vi "GetALL_TAGs.vi"(8 "error in (no error)":errorcluster, 11 "FAMM in":refnum<class "FAMM.lvclass">) -> (0 "error out":errorcluster, 2 "TAGs":string[](array[string]), 3 "FAMM out":refnum<class "FAMM.lvclass">)   [LabVIEW 2014, in "FAMM.lvclass"]
doc: "Read all TAGs"
uses:
  FAMM.lvclass
  FAMM.lvclass/FAMM.ctl
  Common/controls/GlobalClassRefs.vi
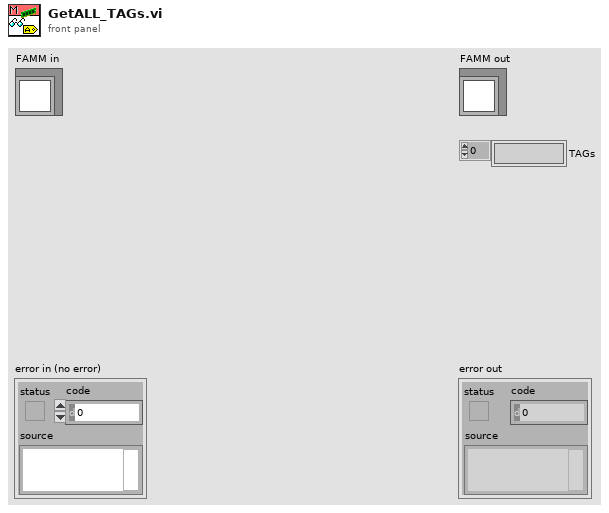
[diagram p1: front panel]
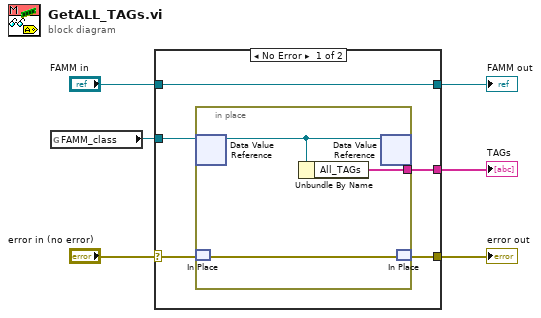
[diagram p0: block diagram]
diagram:
  n1 = global read "GlobalClassRefs.vi" "FAMM_class"() -> (w1:refnum<data-value>)
  n2 = case shown="No Error" "error in (no error)" {
    selector: "error in (no error)" -> [w9 w15]
    tunnel: [w8 w15] -> w5
    tunnel: [w11 w16] -> w3
    tunnel: "FAMM in" -> [w11 w16]
    tunnel: [w10 _] -> w2
    tunnel: w1 -> [w7 _]
    frame No Error {
      n3 = in-place {
        in-place-border: [w14] -> w10
        n4 = in-place-dvr #1(w7) -> (w12:refnum<class "FAMM.lvclass">)  [unwired: 1 out]
        n5 = in-place-match #2(w9) -> (w13:errorcluster)
        n6 = Unbundle By Name(w12) -> ("All_TAGs"=w14:string[])
        n7 = in-place-dvr #1(w12) -> ()  [unwired: 2 out]
        n8 = in-place-match #2(w13) -> (w8:errorcluster)
      }
    }
    frame Error {
    }
  }
  "error out" <- w5
  "FAMM out" <- w3
  "TAGs" <- w2
